vi "Find Item.vi"(7 "$Path or Item Name":string, 8 "error in (no error)":errorcluster, 10 "Offset":i32, 11 "JSON":string) -> (0 "error out":errorcluster, 1 "<JSON>":string caption="<JSON>Item", 2 "Item offset":i32, 3 "Found":bool)   [LabVIEW 2020, in "JSONtext.lvlib"]
doc: "Find the JSON item at the JSON Path specified.\n\nPaths specify an item in a tree of nested Objects, and start with $.\nExample JSON:\n{\"A\":{\"A1\":123,\"A2\":4},\"B\":\"Hi\"}\nAt path $.A.A1 is 123\nAt path $.B (or just B) is \"Hi\"\nAt path $.A (or just A) is {\"A1\":123,\"A2\":4}"
uses:
  <vilib>/JDP Science/JSONtext/JSONtext.lvlib
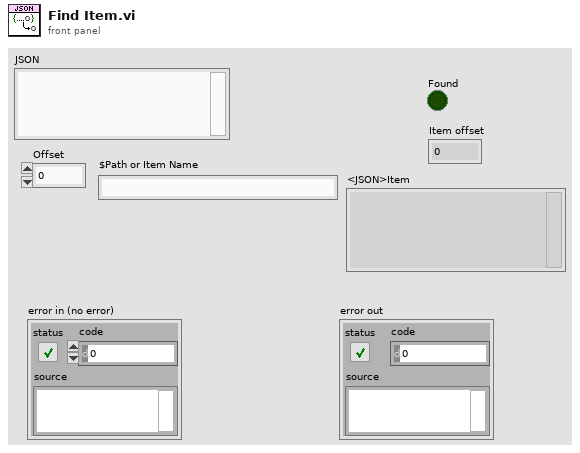
[diagram p1: front panel]
types:
  T1 = typedef "JSONtext.lvlib/JSON Value Type.ctl" = enum16{"Not a JSON Value", "JSON Object", "JSON Array", "String", "Number", "true", "false", "null"}
  T2 = typedef "JSONtext.lvlib/Found Items.ctl" = cluster{"Item offset":i32, "Offset past Item":i32, "Name offset":i32, "Offset past Name":i32, "Found":bool, "Item Type":T3, "Item Index":i32, "Start Offset":i32, "Comma Needed For Insert":T4}
  T3 = typedef "JSONtext.lvlib/Parsing State.ctl" = enum16{"Parser Error", "Object", "Array", "String", "Number/Other", "Leading Whitespace", "Object end", "Array end", "Value end"}
  T4 = typedef "JSONtext.lvlib/Comma Needed for Insert.ctl" = enum8{"False", "True", "Following"}
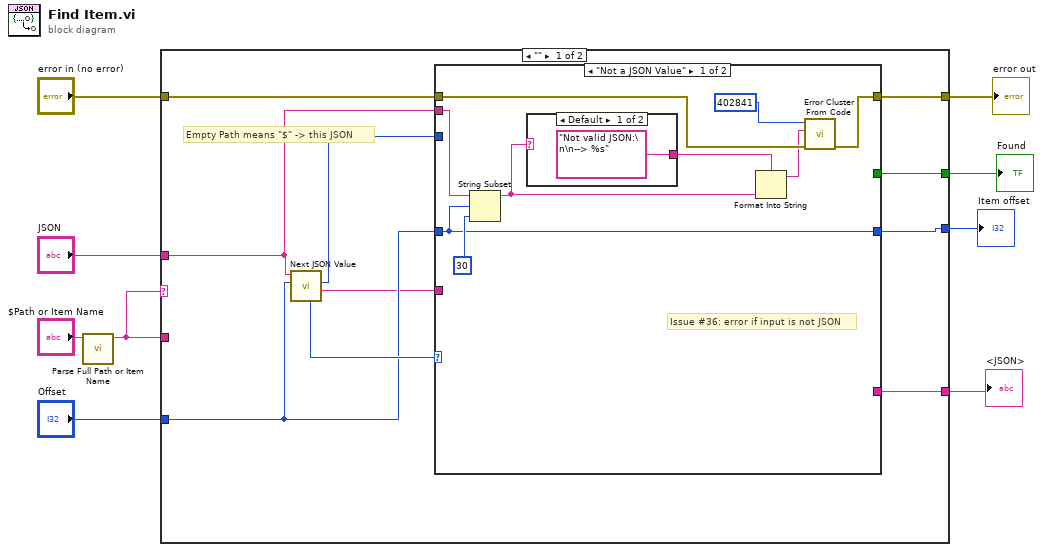
[diagram p0: block diagram]
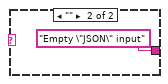
[diagram p2: hidden frame]
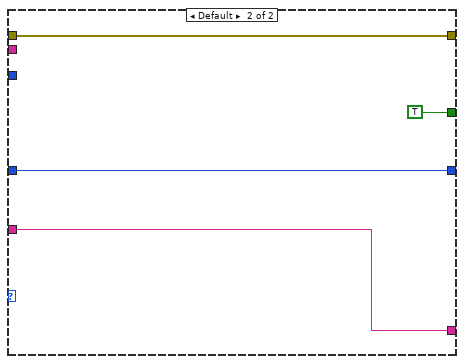
[diagram p3: hidden frame]
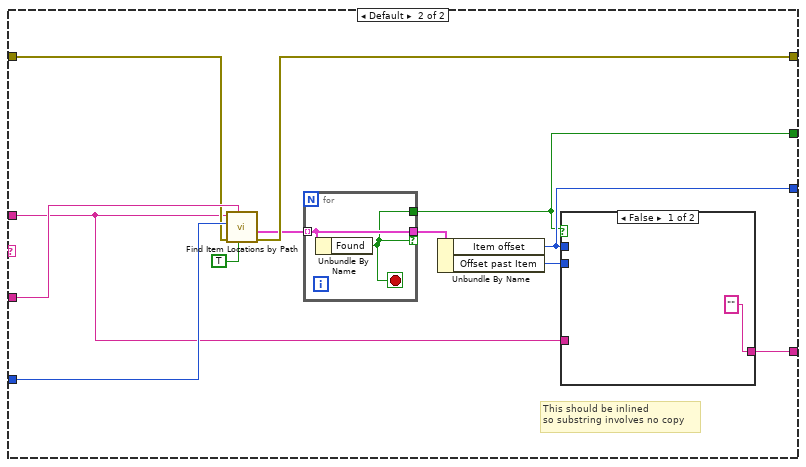
[diagram p4: hidden frame]
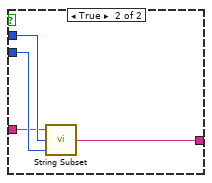
[diagram p5: hidden frame]
diagram:
  n1 = call <vilib>:"Parse Full Path or Item Name.vi"("Full Path (with $) or Name"="$Path or Item Name") -> ("Relative Path or JSON-format name"=w2:string)  [unwired: 10 in]
  n2 = case shown="\"\"" w2 {
    tunnel: w2 -> [_ w46]
    tunnel: "Offset" -> [w17 w45]
    tunnel: "error in (no error)" -> [w13 w44]
    tunnel: [w12 w43] -> w7
    tunnel: "JSON" -> [w11 w42]
    tunnel: [w18 w38] -> w5
    tunnel: [w16 w35] -> w4
    tunnel: [w15 w36] -> w3
    frame "" {
      # "Empty Path means \"$\" -> this JSON"
      n3 = call <vilib>:"Next JSON Value.vi"("Offset"=w17, "JSON"=w11) -> ("<JSON>"=w14:string, "Offset past"=w10:i32, "JSON Value Type"=w19:T1)  [unwired: 6 in, 1 out]
      n4 = case shown="\"Not a JSON Value\"" w19 {
        tunnel: [w21 w34] -> w18
        tunnel: w17 -> [w21 w34]
        tunnel: [_ TRUE ("Found")] -> w16
        tunnel: [_ w32] -> w15
        tunnel: w14 -> [_ w32]
        tunnel: w13 -> [w27 w31]
        tunnel: [w28 w31] -> w12
        tunnel: w11 -> [w25 _]
        tunnel: w10 -> [_ _]
        frame "Not a JSON Value" {
          # "Issue #36: error if input is not JSON"
          n5 = String Subset(string=w25, offset (0)=w21, length (rest)=30 ("length (rest)")) -> (substring=w20:string)
          n6 = case shown="Default" w20 {
            tunnel: ["Not valid JSON:\n\n--> %s" ("format string") "Empty \"JSON\" input" ("format string")] -> w23
            frame Default {
            }
            frame "" {
            }
          }
          n7 = Format Into String(format string=w23, w20) -> (resulting string=w22:string)  [unwired: 2 in, 1 out]
          n8 = call <vilib>:"Error Cluster From Code.vi"("error in (no error)"=w27, "error message (\"\")"=w22, "error code (402840+)"=402841) -> ("error out"=w28:errorcluster)  [unwired: 6 in]
        }
        frame Default {
        }
      }
    }
    frame Default {
      # "This should be inlined\nso substring involves no copy"
      n9 = call <vilib>:"Find Item Locations by Path.vi"("Only return first found"=TRUE, "Path"=w46, "error in (no error)"=w44, "Offset"=w45, "JSON"=w42) -> ("error out"=w43:errorcluster, "Items"=w40:T2[])  [unwired: 5 in]
      n10 = for {
        tunnel: w40 -> [w48] mode=indexing
        tunnel: [w48] -> w39 if=w47
        tunnel: [w47] -> w35
        stop <- w47 stop-if-true
        n11 = Unbundle By Name(w48) -> ("Found"=w47:bool)
      }
      n12 = Unbundle By Name(w39) -> ("Item offset"=w38:i32, "Offset past Item"=w37:i32)
      n13 = case shown="False" w35 {
        tunnel: w42 -> [_ w50]
        tunnel: ["" ("substring") w53] -> w36
        tunnel: w38 -> [_ w52]
        tunnel: w37 -> [_ w51]
        frame False {
        }
        frame True {
          n14 = call <vilib>:"String Subset.vi"("Offset past End"=w51, "Start offset"=w52, "JSON"=w50) -> ("substring"=w53:string)  [unwired: 2 in]
        }
      }
    }
  }
  "error out" <- w7
  "<JSON>" <- w3
  "Found" <- w4
  "Item offset" <- w5
